vi "channel qualification test.vi"() -> (0 "no err":errorcluster, 3 "qualified channels OK":bool)   [LabVIEW 2013, in "CVT tests.lvlib"]
uses:
  CVT tests.lvlib
  <vilib>/NI/Tag Bus Module Framework/channel/channel classification.ctl
  configuration/CVT configuration.lvclass
  <vilib>/NI/Configuration Framework/serializable configuration/NISE_CEF_serializable configuration.lvclass/NISE_CEF_serializable configuration.ctl
  <vilib>/NI/Tag Bus/tag/tag descriptor.lvclass/tag descriptor.ctl
  configuration/CVT configuration.lvclass/CVT configuration.ctl
  <vilib>/NI/Configuration Framework/serializable configuration/Read UID.vi
  configuration/Write channels.vi
  <vilib>/Utility/LVClass/Get LV Class Name.vi
  <vilib>/NI/Configuration Framework/error generator/NISE_error generator.vi
  <vilib>/NI/Tag Bus Module Framework/channel/TBM channel.lvclass
  <vilib>/NI/Tag Bus/tag/tag descriptor.lvclass
  <vilib>/NI/Tag Bus Module Framework/module configuration/TBM module configuration.lvclass
  <vilib>/NI/Configuration Framework/serializable configuration/NISE_CEF_serializable configuration.lvclass
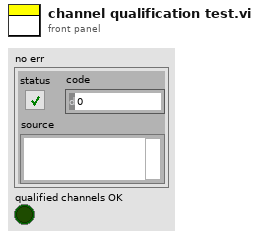
[diagram p1: front panel]
types:
  T1 = typedef "TBM channel.lvclass/channel classification.ctl" = enum16{"input data", "output data", "processing parameter", "processing result"}
  T2 = typedef "tag bus.lvlib/tag descriptor.lvclass/Data Type.ctl" = enum16{"Double", "Single", "I64", "I32", "I16", "I8", "U64", "U32", "U16", "U8", "Boolean", "String", "Array of Double", "Array of Single", "Array of I64", "Array of I32", "Array of I16", "Array of I8", "Array of U64", "Array of U32", "Array of U16", "Array of U8", "Array of Boolean", "Array of String"}
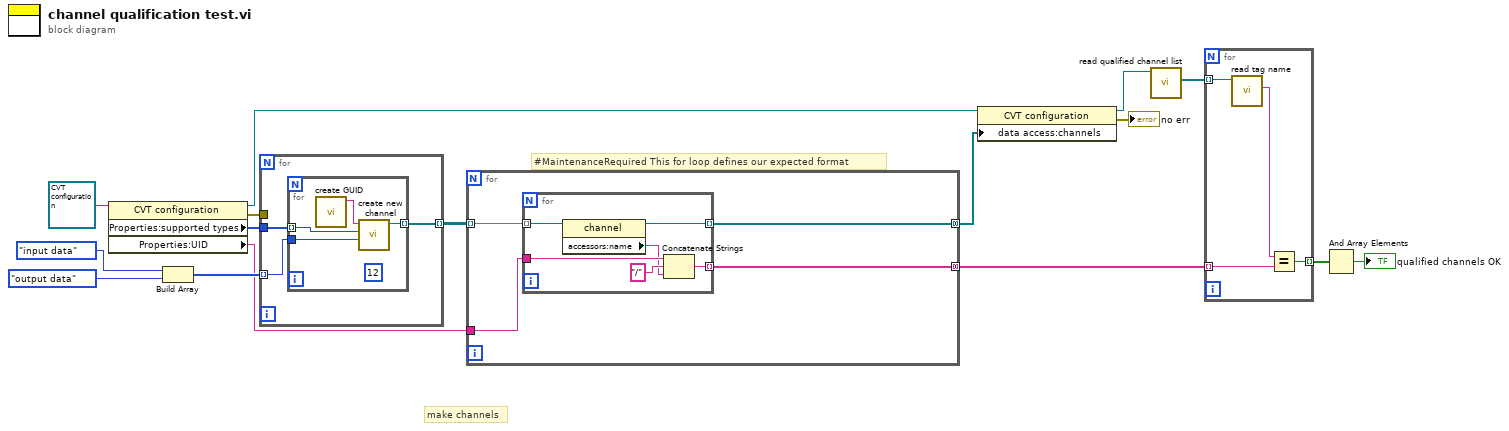
[diagram p0: block diagram]
diagram:
  # "#MaintenanceRequired This for loop defines our expected format"
  # "make channels"
  n1 = property class="CVT configuration"(reference=refnum<class "CVT configuration.lvclass"> refnum ("tag bus configurable plugin module configuration")) -> (reference out=w13:refnum<class "CVT configuration.lvclass">, error out=w1:errorcluster, "Properties:supported types"=w12:T2[], "Properties:UID"=w2:string)  [unwired: 1 in]
  n2 = Build Array(channel_classification."input data" ("channel classification"), channel_classification."output data" ("channel classification")) -> (w14:T1[])
  n3 = for {
    tunnel: w14 -> [w19] mode=indexing
    tunnel: [w17] -> w11 mode=indexing
    tunnel: w12 -> [w18]
    tunnel: w1 -> [_]
    n4 = for {
      tunnel: w19 -> [w22]
      tunnel: [w23] -> w17 mode=indexing
      tunnel: w18 -> [w21] mode=indexing
      (unwired) 12
      n5 = call <vilib>:"create GUID.vi"() -> ("uuid"=w20:string)  [unwired: 10 in, 1 out]
      n6 = call <vilib>:"create new channel.vi"("channel classification"=w22, "data type"=w21, "channel name"=w20) -> ("channel"=w23:refnum<class "TBM channel.lvclass">)  [unwired: 8 in]
    }
  }
  n7 = for {
    tunnel: [w27] -> w3 mode=concatenating
    tunnel: w11 -> [w26] mode=indexing
    tunnel: w2 -> [w25]
    tunnel: [w24] -> w7 mode=concatenating
    n8 = for {
      tunnel: [w28] -> w27 mode=indexing
      tunnel: w26 -> [w33] mode=indexing
      tunnel: w25 -> [w32]
      tunnel: [w29] -> w24 mode=indexing
      n9 = property class="channel"(reference=w33) -> (reference out=w28:refnum<class "TBM channel.lvclass">, "accessors:name"=w30:string)  [unwired: 1 in, 1 out]
      n10 = Concatenate Strings(w32, "/" ("string"), w30) -> (w29:string)
    }
  }
  n11 = property class="CVT configuration"(reference=w13, "data access:channels"=w3) -> (reference out=w4:refnum<class "CVT configuration.lvclass">, error out=→"no err":errorcluster)  [unwired: 1 in]
  n12 = call <vilib>:"read qualified channel list.vi"("module configuration in"=w4) -> ("qualified channels"=w8:refnum<class "TBM channel.lvclass">[])  [unwired: 9 in, 1 out]
  n13 = for {
    tunnel: w7 -> [w36] mode=indexing
    tunnel: w8 -> [w37] mode=indexing
    tunnel: [w34] -> w10 mode=indexing
    n14 = call <vilib>:"read tag name.vi"("system tag in"=w37) -> ("name"=w35:string)  [unwired: 8 in, 2 out]
    n15 = Equal?(x=w35, y=w36) -> (x = y?=w34:bool)
  }
  n16 = And Array Elements(Boolean array=w10) -> (logical AND=→"qualified channels OK":bool)
